vi "0MAIN_v1.vi"() -> ()   [LabVIEW 2021]
uses:
  <vilib>/Instr/_visa.llb/VISA Open Access Mode.ctl
  <vilib>/Instr/_visa.llb/VISA Configure Serial Port (Instr).vi
panel:
  out "LF2":bool
  out "LF1":bool
  out "Пересчитано":bool=TRUE
  out "Метка получена 2":bool
  out "Время старта":string
  out "Ошибка файла":errorcluster
  out "Метка получена":bool
  out "Файл данных":refnum<file>
  out "Файл журнала":refnum<file>
  out "Номер метки":bool=TRUE
  out "error out 2":errorcluster
  in  "Управление":enum32{"Отладка", "График", "Настройки"}(tab)
  in  "Пересчитать в частоты":bool
  in  "Частота метки 2":bool
  in  "Записать данные":bool
  in  "Очистка буфера":bool
  in  "Чтение данных":bool
  in  "Установить":string
  in  "Отправка":bool
  out "Данные с МК":string
  out "Развертка X (В/ГГц)":dbl[](array[numeric])
  out "Сигнал Y (В)":dbl[](array[numeric])
  out "Метки (В, ГГц)":dbl[][](array[numeric])
  in  "Частота метки":bool
  in  "Выход":bool
  in  "Расчет графика":bool
  out "График":T1(graph)
  in  "Путь к файлу данных":path
  in  "Путь к логу":path
  in  "Логирование":bool
  out "Ошибка":T2
  in  "Порт":refnum<visa-resource-name>
  in  "Скорость передачи (9600)":u32=9600
  in  "Символ окончания (\\n)":u8=10 format="%.0x"
  in  "Режим доступа":T3 items=["VISA Defaults"=0, "Exclusive Lock"=1, "Load Configured Settings"=4]
  in  "Бит данных (8)":u8=8 format="%.0x"
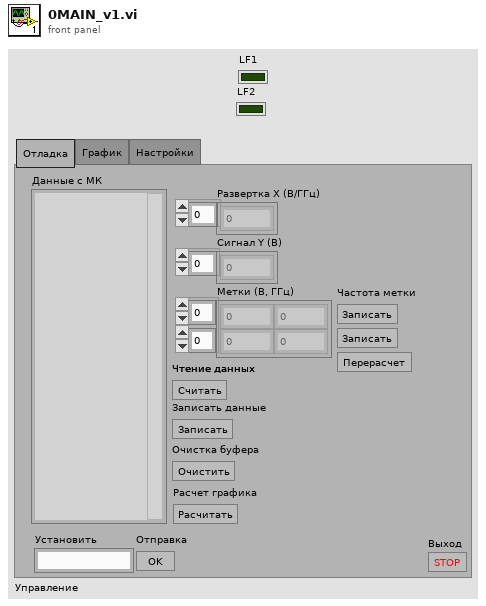
[diagram p1: front panel]
types:
  T1 = cluster{"Развертка X (В)":dbl[], "Сигнал Y (В)":dbl[]}
  T2 = cluster{"Статус":bool, "Код":i32, "Источник":string}
  T3 = typedef "VISA Open Access Mode.ctl" = u32
  T4 = enum16{"open", "replace", "create", "open or create", "replace or create", "replace or create with confirmation"}
  T5 = typedef "NI_Matrix.lvlib/RealMatrix.ctl" = dbl[][]
  T6 = cluster{"Развертка X (В/ГГц)":dbl[], "Сигнал Y (В)":dbl[]}
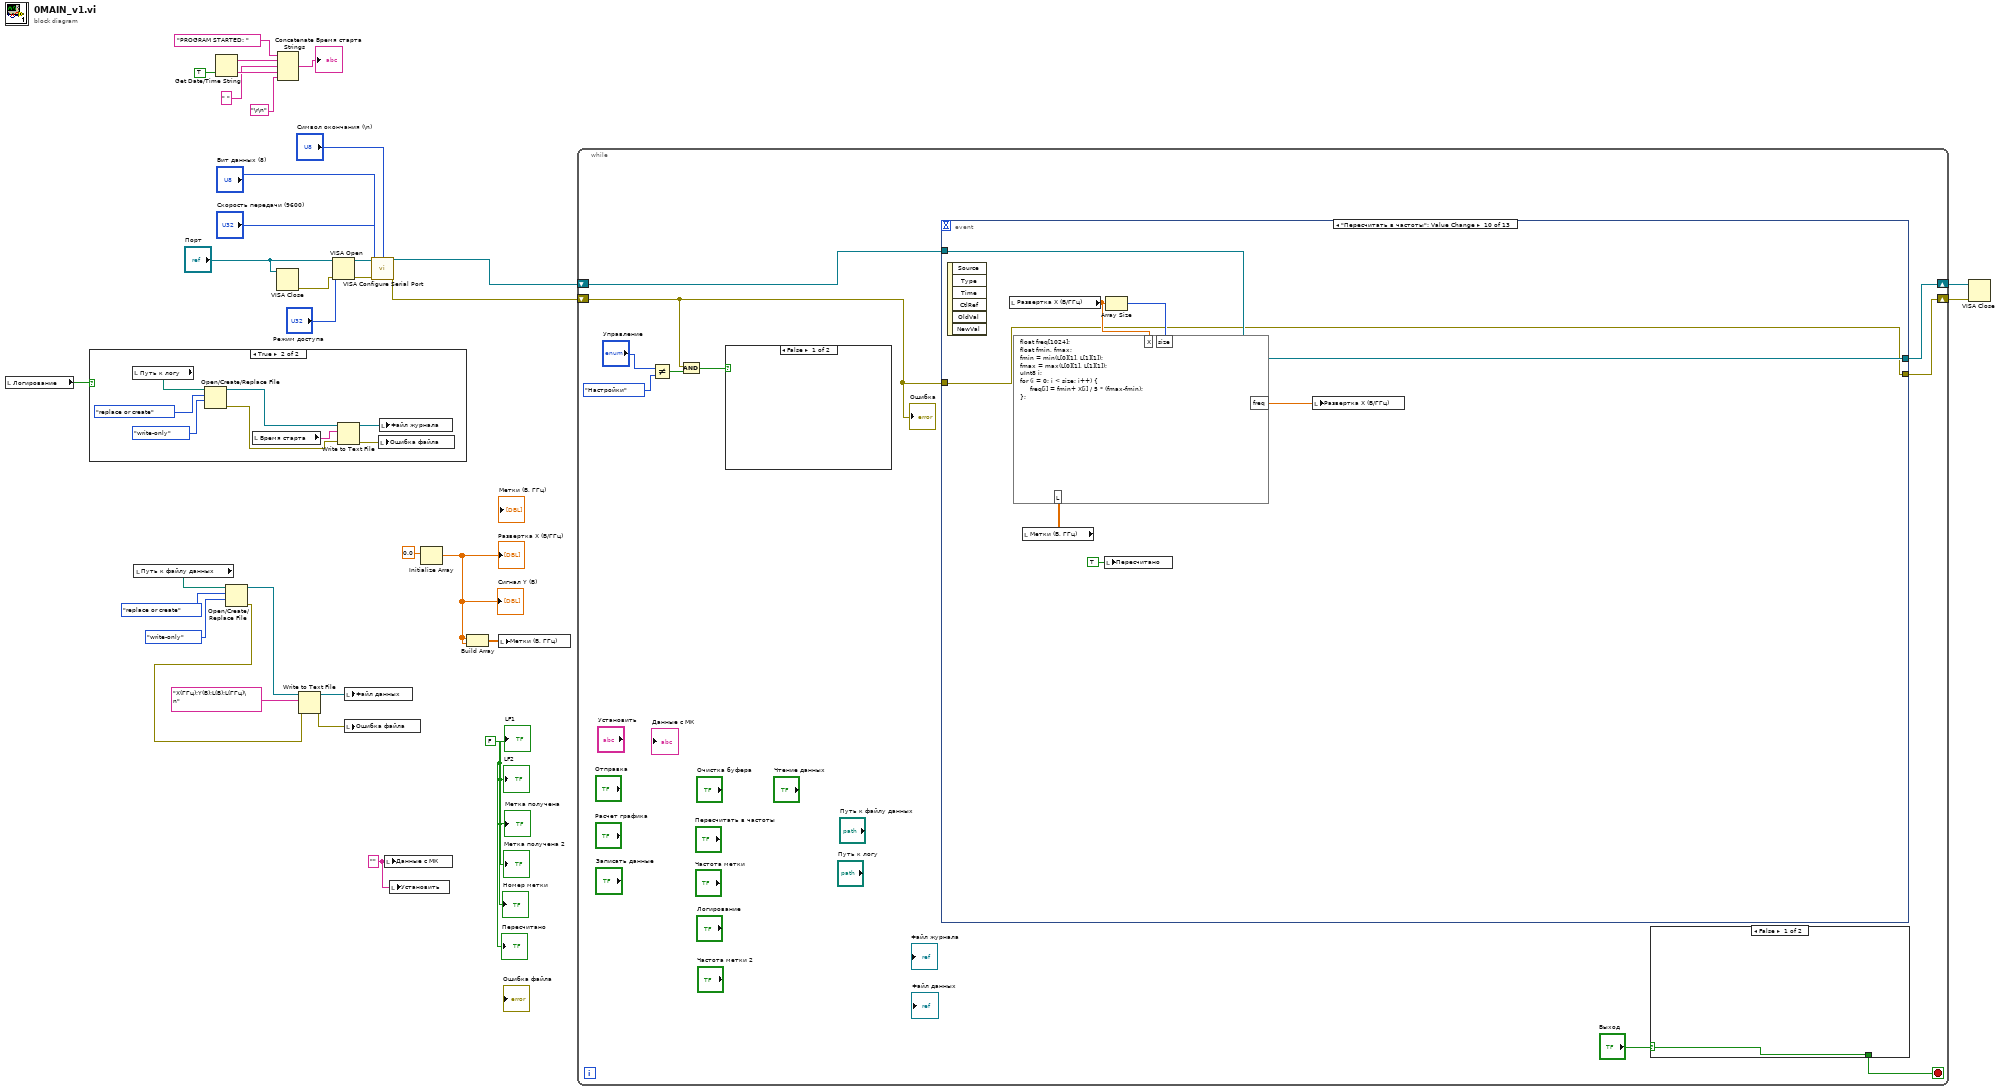
[diagram p0: block diagram]
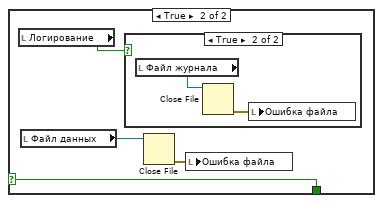
[diagram p3: hidden frame]
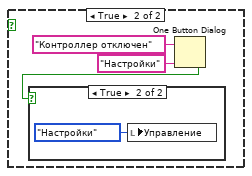
[diagram p5: hidden frame]
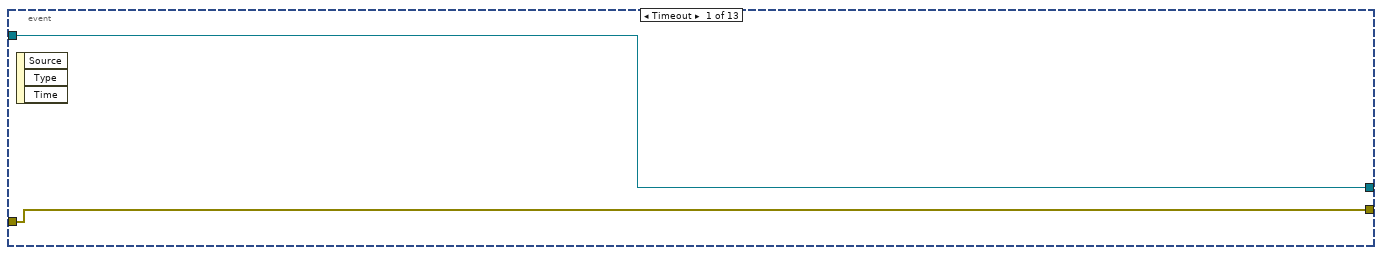
[diagram p7: hidden frame]
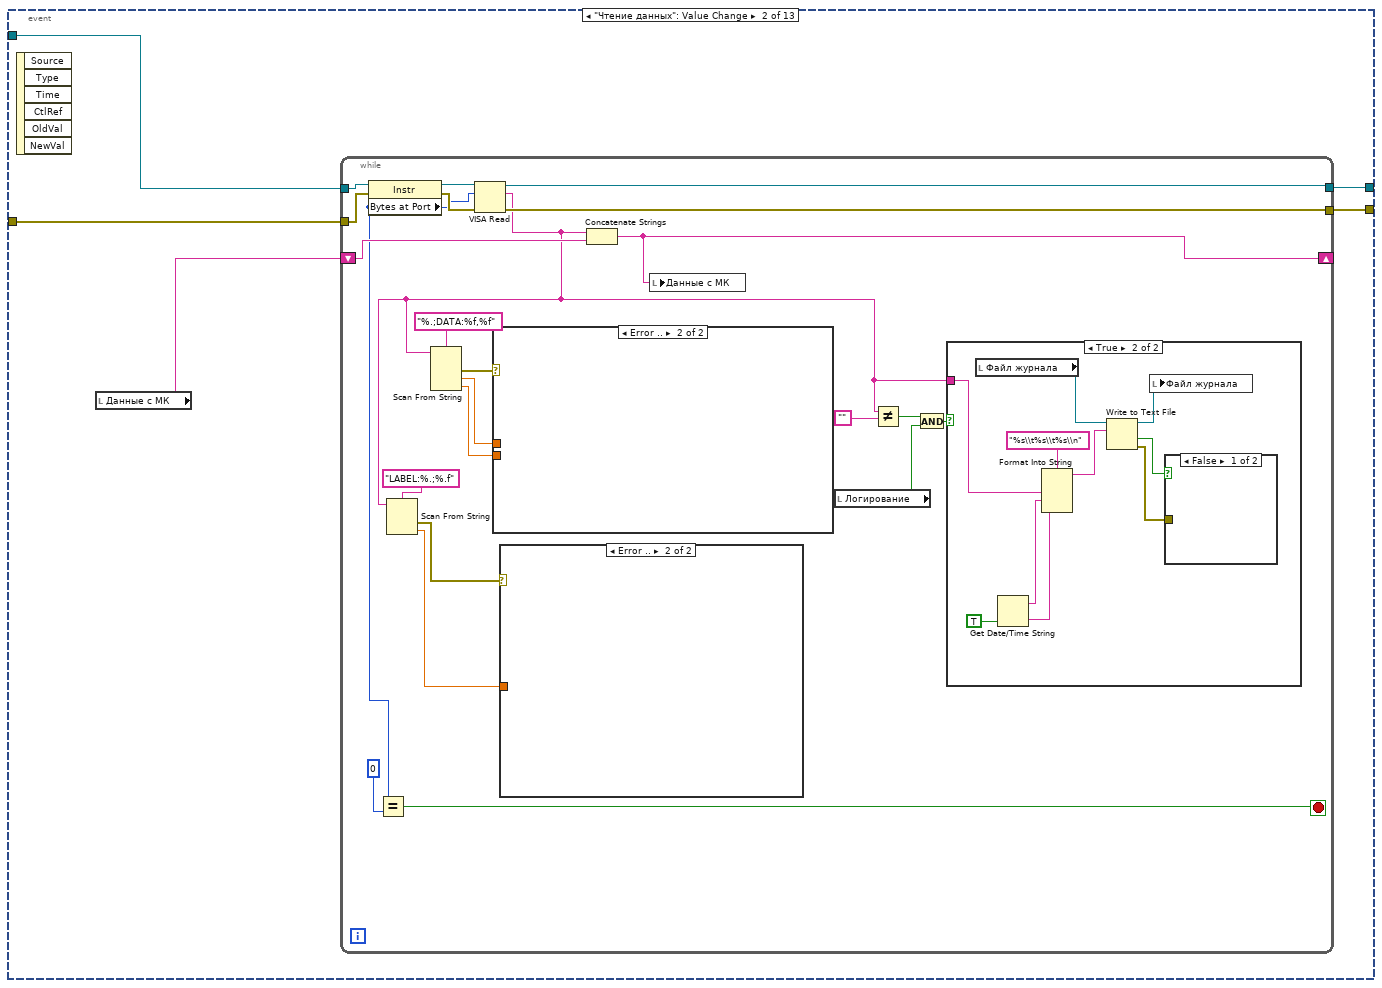
[diagram p8: hidden frame]
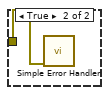
[diagram p10: hidden frame]
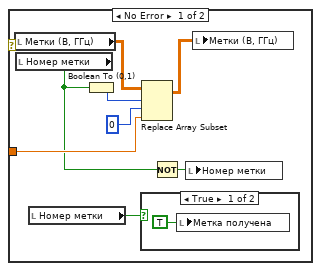
[diagram p11: hidden frame]
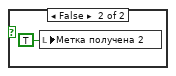
[diagram p12: hidden frame]
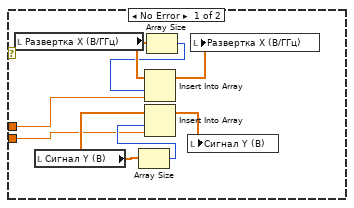
[diagram p13: hidden frame]
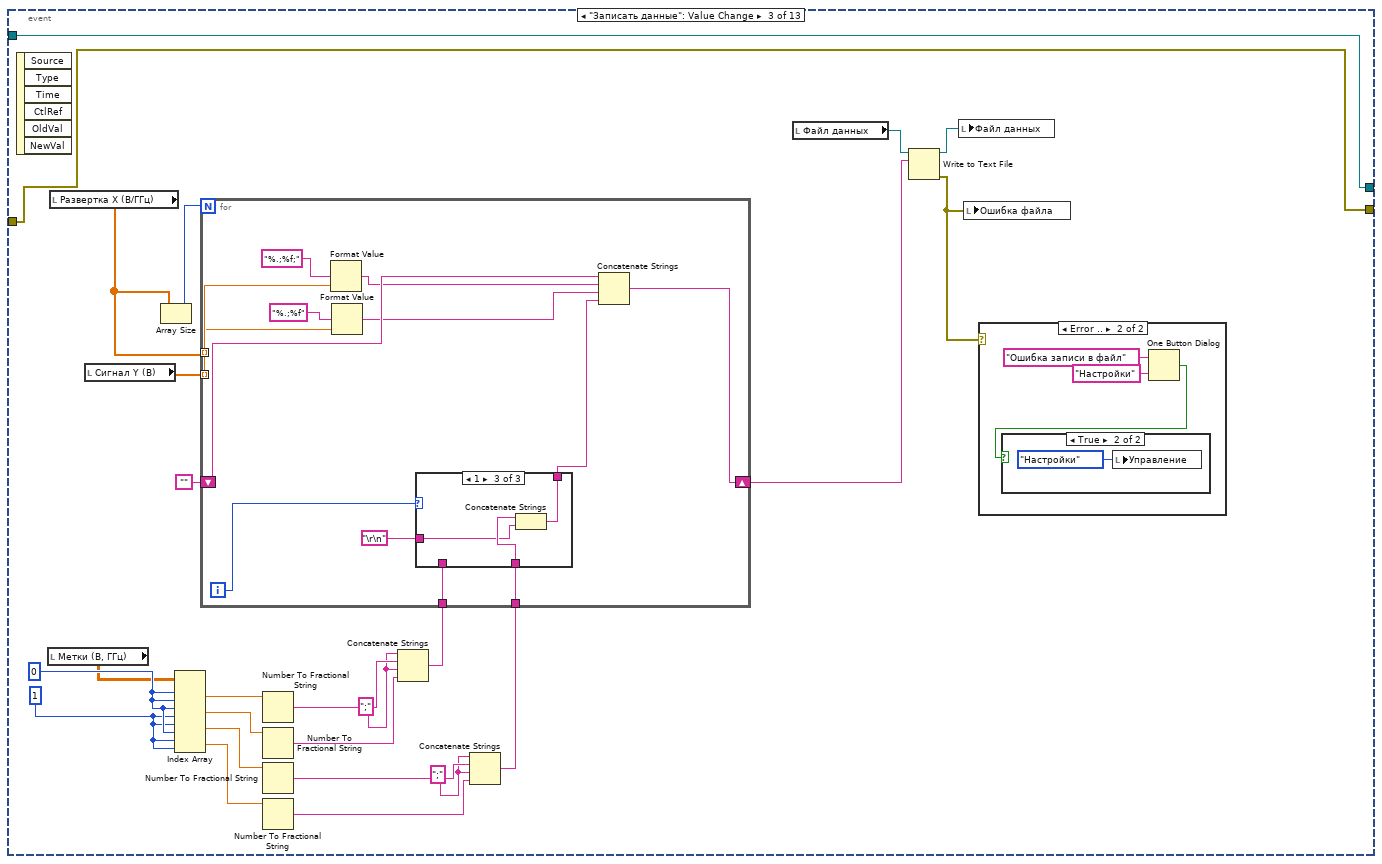
[diagram p14: hidden frame]
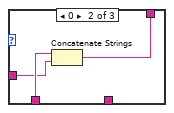
[diagram p18: hidden frame]
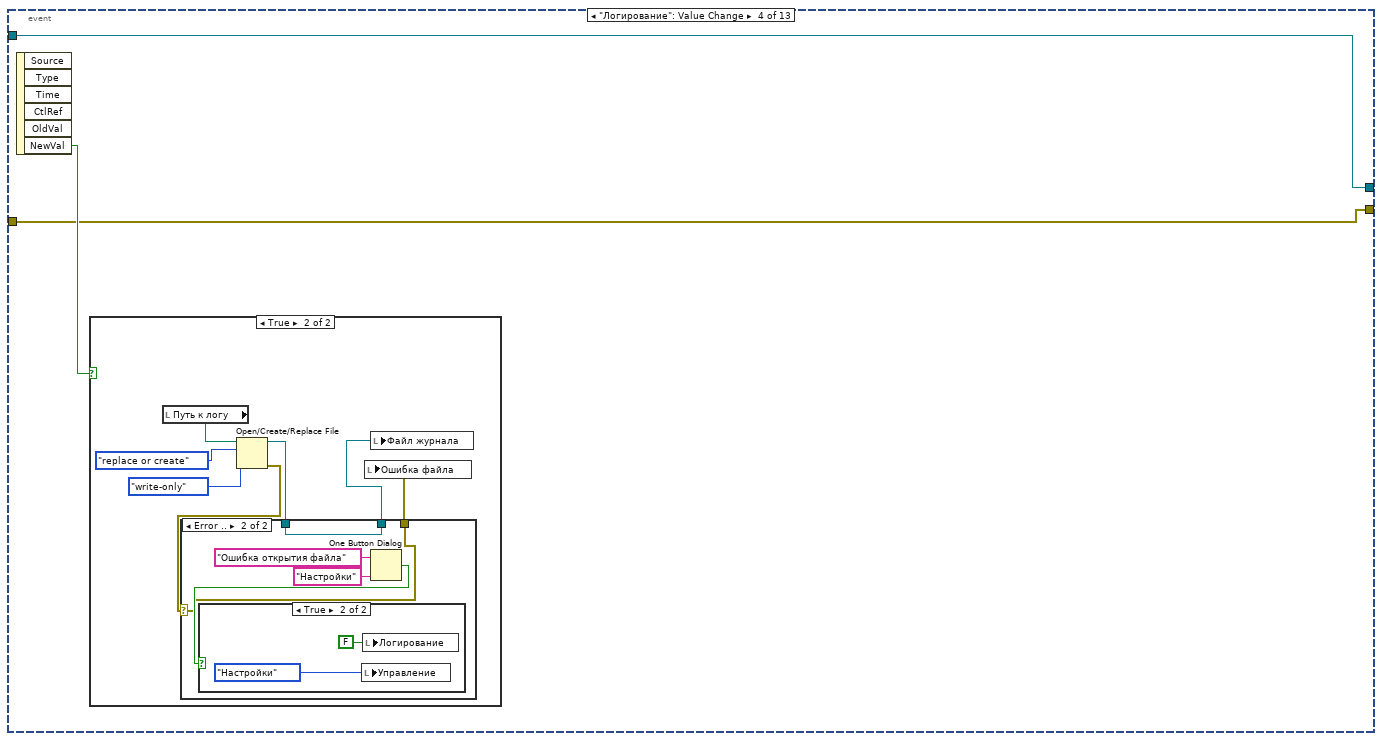
[diagram p19: hidden frame]
diagram:
  w1 = "" ("Данные с МК")
  w2 = FALSE ("Частоты определены")
  n1 = local read "Логирование"() -> (w13:bool)
  n2 = case shown="True" w13 {
    frame False {
    }
    frame True {
      n3 = local read "Путь к логу"() -> (w41:path)
      n4 = Open/Create/Replace File(file path (use dialog)=w41, operation (0:open)=T4."replace or create", access (0:read/write)=enum16{"read/write", "read-only", "write-only"}."write-only") -> (refnum out=w34:refnum<file>, error out=w35:errorcluster)  [unwired: 3 in, 1 out]
      n5 = local read "Время старта"() -> (w36:string)
      n6 = Write to Text File(file (use dialog)=w34, text=w36, error in=w35) -> (refnum out=w37:refnum<file>, error out=w38:errorcluster)  [unwired: 1 in, 1 out]
      n7 = local write "Ошибка файла"(w38) -> ()
      n8 = local write "Файл журнала"(w37) -> ()
    }
  }
  n9 = local read "Путь к файлу данных"() -> (w18:path)
  n10 = Get Date/Time String(want seconds? (F)=TRUE) -> (date string=w12:string, time string=w4:string)  [unwired: 2 in]
  n11 = Open/Create/Replace File(file path (use dialog)=w18, operation (0:open)=T4."replace or create", access (0:read/write)=enum16{"read/write", "read-only", "write-only"}."write-only") -> (refnum out=w6:refnum<file>, error out=w7:errorcluster)  [unwired: 3 in, 1 out]
  n12 = VISA Close(VISA resource name="Порт") -> (error out=w19:errorcluster)  [unwired: 1 in]
  n13 = Concatenate Strings("PROGRAM STARTED: " ("string"), w12, " ", w4, "\r\n" ("string")) -> (→"Время старта":string)
  n14 = Write to Text File(file (use dialog)=w6, text="X(ГГц);Y(В);L(В);L(ГГц)\n", error in=w7) -> (refnum out=w9:refnum<file>, error out=w10:errorcluster)  [unwired: 1 in, 1 out]
  n15 = VISA Open(access mode="Режим доступа", error in (no error)=w19, VISA resource name="Порт") -> (VISA resource name=w30:refnum<visa-resource-name>, error out=w29:errorcluster)  [unwired: 2 in]
  n16 = local write "Файл данных"(w9) -> ()
  n17 = local write "Ошибка файла"(w10) -> ()
  n18 = call-poly "VISA Configure Serial Port"("VISA resource name"=w30, "termination char\n(0xA = '\\n' = LF)"="Символ окончания (\\n)", "baud rate (9600)"="Скорость передачи (9600)", "data bits (8)"="Бит данных (8)", "error in (no error)"=w29) -> ("VISA resource name out"=w24:refnum<visa-resource-name>, "error out"=w26:errorcluster)  [unwired: 9 in]
  n19 = local write "Данные с МК"(w1) -> ()
  n20 = local write "Установить"(w1) -> ()
  n21 = Initialize Array(0.0 ("element")) -> (w21:dbl[])  [unwired: 1 in]
  "Развертка X (В/ГГц)" <- w21
  "Сигнал Y (В)" <- w21
  n22 = Build Array(w21, w21) -> (w20:T5)
  n23 = local write "Метки (В, ГГц)"(w20) -> ()
  n24 = while {
    shift-right: [w43] -> w25
    shift-left: w26 -> [w47]
    shift-right: [w42] -> w23
    shift-left: w24 -> [w51]
    stop <- w44 stop-if-true
    n25 = Not Equal?(x="Управление", y=enum32{"Отладка", "График", "Настройки"}."Настройки" ("Tab Control")) -> (x != y?=w48:bool)
    n26 = And(x=w47, y=w48) -> (x .and. y?=w46:bool)
    n27 = case shown="False" w46 {
      frame False {
      }
      frame True {
        n28 = One Button Dialog(message="Контроллер отключен", button name ("OK")="Настройки") -> (true=w60:bool)
        n29 = case shown="True" w60 {
          frame False {
          }
          frame True {
            n30 = local write "Управление"(enum32{"Отладка", "График", "Настройки"}."Настройки" ("Tab Control")) -> ()
          }
        }
      }
    }
    n31 = event shown="[9] \"Пересчитать в частоты\": Value Change" {
      selector: _ -> [_ _ _ _ _ _ _ _ _ _ _ _ _]
      dyn-events: _ -> [_ _ _ _ _ _ _ _ _ _ _ _ _]
      timeout: _ -> [_ _ _ _ _ _ _ _ _ _ _ _ _]
      tunnel: w47 -> [w64 w69 w122 w172 w193 _ w208 w218 w232 w237 w244 w269 w281]
      tunnel: [w64 w68 w122 w172 w193 w198 w208 w218 w232 w237 w244 w269 w280] -> w43
      tunnel: w51 -> [w63 w67 w123 w171 w194 _ w207 w219 w233 w238 w245 w270 w279]
      tunnel: [w63 w66 w123 w171 w194 w202 w207 w219 w233 w238 w245 w270 w278] -> w42
      event Timeout {
        n32 = event-data() -> ()  [unwired: 1 in, 3 out]
      }
      event "Чтение данных": Value Change {
        n33 = event-data() -> ()  [unwired: 1 in, 6 out]
        n34 = local read "Данные с МК"() -> (w65:string)
        n35 = while {
          tunnel: w67 -> [w87]
          tunnel: w69 -> [w86]
          tunnel: [w92] -> w66
          tunnel: [w91] -> w68
          shift-right: [w75] -> _
          shift-left: w65 -> [w90]
          stop <- w85 stop-if-true
          n36 = property class="Instr"(reference=w87, error in=w86) -> (reference out=w89:refnum<visa-resource-name>, error out=w88:errorcluster, "Bytes at Port"=w83:u32)
          n37 = Equal?(x=w83, y=u32 0 ("x")) -> (x = y?=w85:bool)
          n38 = VISA Read(VISA resource name=w89, byte count=w83, error in (no error)=w88) -> (VISA resource name out=w92:refnum<visa-resource-name>, read buffer=w71:string, error out=w91:errorcluster)  [unwired: 1 out]
          n39 = Scan From String(format string="LABEL:%.;%.f", input string=w71) -> (error out=w79:errorcluster, output 1=w78:dbl)  [unwired: 3 in, 2 out]
          n40 = Scan From String(format string="%.;DATA:%f,%f", input string=w71) -> (error out=w76:errorcluster, output 1=w82:dbl, output 2=w81:dbl)  [unwired: 4 in, 2 out]
          n41 = case shown="Error .." w76 {
            tunnel: w82 -> [w117 _]
            tunnel: w81 -> [w116 _]
            frame No Error {
              n42 = local read "Развертка X (В/ГГц)"() -> (w121:dbl[])
              n43 = local read "Сигнал Y (В)"() -> (w120:dbl[])
              n44 = Array Size(array=w120) -> (size(s)=w119:i32)
              n45 = Insert Into Array(array=w120, index=w119, new element=w116) -> (w114:dbl[])
              n46 = Array Size(array=w121) -> (size(s)=w118:i32)
              n47 = Insert Into Array(array=w121, index=w118, new element=w117) -> (w115:dbl[])
              n48 = local write "Сигнал Y (В)"(w114) -> ()
              n49 = local write "Развертка X (В/ГГц)"(w115) -> ()
            }
            frame Error {
            }
          }
          n50 = case shown="Error .." w79 {
            tunnel: w78 -> [w108 _]
            frame No Error {
              n51 = local read "Метки (В, ГГц)"() -> (w110:dbl[][])
              n52 = local read "Номер метки"() -> (w105:bool)
              n53 = local read "Номер метки"() -> (w104:bool)
              n54 = Boolean To (0,1)(Boolean=w105) -> (0, 1=w109:i16)
              n55 = case shown="True" w104 {
                frame True {
                  n56 = local write "Метка получена"(TRUE ("Метка получена")) -> ()
                }
                frame False {
                  n57 = local write "Метка получена 2"(TRUE ("Метка получена")) -> ()
                }
              }
              n58 = Replace Array Subset(array=w110, new element=w108, index (row)=w109, index (col)=0 ("disabled index (col)")) -> (w111:T5)
              n59 = Not(x=w105) -> (.not. x?=w106:bool)
              n60 = local write "Номер метки"(w106) -> ()
              n61 = local write "Метки (В, ГГц)"(w111) -> ()
            }
            frame Error {
            }
          }
          n62 = Concatenate Strings(w71, w90) -> (w75:string)
          n63 = local write "Данные с МК"(w75) -> ()
          n64 = local read "Логирование"() -> (w70:bool)
          n65 = Not Equal?(x=w71, y="") -> (x != y?=w73:bool)
          n66 = And(x=w73, y=w70) -> (x .and. y?=w74:bool)
          n67 = case shown="True" w74 {
            tunnel: w71 -> [_ w93]
            frame False {
            }
            frame True {
              n68 = local read "Файл журнала"() -> (w98:refnum<file>)
              n69 = Get Date/Time String(want seconds? (F)=TRUE) -> (date string=w97:string, time string=w96:string)  [unwired: 2 in]
              n70 = Format Into String(format string="%s\\t%s\\t%s\\n", w93, w97, w96) -> (resulting string=w94:string)  [unwired: 2 in, 1 out]
              n71 = Write to Text File(file (use dialog)=w98, text=w94) -> (refnum out=w99:refnum<file>, cancelled=w101:bool, error out=w100:errorcluster)  [unwired: 2 in]
              n72 = local write "Файл журнала"(w99) -> ()
              n73 = case shown="False" w101 {
                tunnel: w100 -> [_ w103]
                frame False {
                }
                frame True {
                  n74 = call <vilib>:"Simple Error Handler.vi"("error in (no error)"=w103) -> ()  [unwired: 4 in, 5 out]
                }
              }
            }
          }
        }
      }
      event "Записать данные": Value Change {
        w128 = ";"
        w129 = ";"
        w140 = 1
        w141 = 0
        n75 = event-data() -> ()  [unwired: 1 in, 6 out]
        n76 = local read "Метки (В, ГГц)"() -> (w127:dbl[][])
        n77 = local read "Развертка X (В/ГГц)"() -> (w144:dbl[])
        n78 = local read "Сигнал Y (В)"() -> (w145:dbl[])
        n79 = Array Size(array=w144) -> (size(s)=w146:i32)
        n80 = Index Array(array=w127, index (row) #1=w141, index (col) #1=w141, index (row) #2=w141, index (col) #2=w140, index (row) #3=w140, index (col) #3=w141, index (row) #4=w140, index (col) #4=w140) -> (element #1=w139:dbl, element #2=w138:dbl, element #3=w137:dbl, element #4=w136:dbl)
        n81 = Number To Fractional String(number=w139) -> (F-format string=w132:string)  [unwired: 3 in]
        n82 = Number To Fractional String(number=w138) -> (F-format string=w133:string)  [unwired: 3 in]
        n83 = Number To Fractional String(number=w137) -> (F-format string=w134:string)  [unwired: 3 in]
        n84 = Number To Fractional String(number=w136) -> (F-format string=w135:string)  [unwired: 3 in]
        n85 = Concatenate Strings(w128, w132, w128, w133) -> (w131:string)
        n86 = Concatenate Strings(w129, w134, w129, w135) -> (w130:string)
        n87 = for {
          N: w146 -> [_]
          tunnel: w145 -> [w162] mode=indexing
          tunnel: w144 -> [w163] mode=indexing
          shift-right: [w159] -> w126
          shift-left: "" -> [w154]
          tunnel: w131 -> [w157]
          tunnel: w130 -> [w156]
          i -> [w158]
          n88 = Format Value(format string="%.;%f;", value (0)=w163) -> (output string=w153:string)  [unwired: 1 in]
          n89 = Format Value(format string="%.;%f", value (0)=w162) -> (output string=w152:string)  [unwired: 1 in]
          n90 = case shown="1" w158 {
            tunnel: w157 -> [_ w167 _]
            tunnel: w156 -> [_ _ w170]
            tunnel: "\r\n" -> [w164 w166 w169]
            tunnel: [w164 w165 w168] -> w151
            frame Default {
            }
            frame 0 {
              n91 = Concatenate Strings(w167, w166) -> (w165:string)
            }
            frame 1 {
              n92 = Concatenate Strings(w170, w169) -> (w168:string)
            }
          }
          n93 = Concatenate Strings(w154, w153, w152, w151) -> (w159:string)
        }
        n94 = local read "Файл данных"() -> (w143:refnum<file>)
        n95 = Write to Text File(file (use dialog)=w143, text=w126) -> (refnum out=w142:refnum<file>, error out=w124:errorcluster)  [unwired: 2 in, 1 out]
        n96 = local write "Файл данных"(w142) -> ()
        n97 = local write "Ошибка файла"(w124) -> ()
        n98 = case shown="Error .." w124 {
          frame No Error {
          }
          frame Error {
            n99 = One Button Dialog(message="Ошибка записи в файл", button name ("OK")="Настройки") -> (true=w148:bool)
            n100 = case shown="True" w148 {
              frame False {
              }
              frame True {
                n101 = local write "Управление"(enum32{"Отладка", "График", "Настройки"}."Настройки" ("Управление")) -> ()
              }
            }
          }
        }
      }
      event "Логирование": Value Change {
        n102 = event-data() -> ("NewVal"=w173:bool)  [unwired: 1 in, 5 out]
        n103 = case shown="True" w173 {
          frame False {
          }
          frame True {
            n104 = local read "Путь к логу"() -> (w180:path)
            n105 = Open/Create/Replace File(file path (use dialog)=w180, operation (0:open)=T4."replace or create", access (0:read/write)=enum16{"read/write", "read-only", "write-only"}."write-only") -> (refnum out=w178:refnum<file>, error out=w179:errorcluster)  [unwired: 3 in, 1 out]
            n106 = case shown="Error .." w179 {
              selector: w179 -> [w184 w186]
              tunnel: w178 -> [w185 w187]
              tunnel: [w183 w186] -> w177
              tunnel: [w182 w187] -> w176
              frame No Error {
                n107 = local read "Время старта"() -> (w181:string)
                n108 = Write to Text File(file (use dialog)=w185, text=w181, error in=w184) -> (refnum out=w182:refnum<file>, error out=w183:errorcluster)  [unwired: 1 in, 1 out]
              }
              frame Error {
                n109 = One Button Dialog(message="Ошибка открытия файла", button name ("OK")="Настройки") -> (true=w189:bool)
                n110 = case shown="True" w189 {
                  frame False {
                  }
                  frame True {
                    n111 = local write "Управление"(enum32{"Отладка", "График", "Настройки"}."Настройки" ("Управление")) -> ()
                    n112 = local write "Логирование"(FALSE ("Логирование")) -> ()
                  }
                }
              }
            }
            n113 = local write "Ошибка файла"(w177) -> ()
            n114 = local write "Файл журнала"(w176) -> ()
          }
        }
      }
      event "Очистка буфера": Value Change {
        n115 = event-data() -> ()  [unwired: 1 in, 6 out]
        n116 = local write "Данные с МК"("") -> ()
      }
      event "Порт": Value Change {
        n117 = event-data() -> ("OldVal"=w197:refnum<visa-resource-name>, "NewVal"=w206:refnum<visa-resource-name>)  [unwired: 1 in, 4 out]
        n118 = local read "Скорость передачи (9600)"() -> (w201:u32)
        n119 = local read "Бит данных (8)"() -> (w200:u8)
        n120 = local read "Режим доступа"() -> (w205:T3)
        n121 = local read "Символ окончания (\\n)"() -> (w199:u8)
        n122 = VISA Close(VISA resource name=w197) -> (error out=→"error out 2":errorcluster)  [unwired: 1 in]
        n123 = VISA Open(access mode=w205, VISA resource name=w206) -> (VISA resource name=w204:refnum<visa-resource-name>, error out=w203:errorcluster)  [unwired: 3 in]
        n124 = call-poly "VISA Configure Serial Port"("VISA resource name"=w204, "termination char\n(0xA = '\\n' = LF)"=w199, "baud rate (9600)"=w201, "data bits (8)"=w200, "error in (no error)"=w203) -> ("VISA resource name out"=w202:refnum<visa-resource-name>, "error out"=w198:errorcluster)  [unwired: 9 in]
      }
      event "Частота метки": Value Change {
        n125 = event-data() -> ()  [unwired: 1 in, 6 out]
        n126 = local read "Метка получена"() -> (w209:bool)
        n127 = case shown="True" w209 {
          frame False {
          }
          frame True {
            n128 = local read "Установить"() -> (w216:string)
            n129 = local read "Метки (В, ГГц)"() -> (w212:dbl[][])
            n130 = Scan Value(string=w216, format string="%.;%f") -> (value=w217:dbl)  [unwired: 1 in, 1 out]
            n131 = Replace Array Subset(array=w212, new element=w217, index (row)=0 ("disabled index (row)"), index (col)=1 ("disabled index (col)")) -> (w213:T5)
            n132 = local write "Метки (В, ГГц)"(w213) -> ()
            n133 = local write "LF1"(TRUE ("LF1")) -> ()
          }
        }
      }
      event "Частота метки 2": Value Change {
        n134 = event-data() -> ()  [unwired: 1 in, 6 out]
        n135 = local read "Метка получена 2"() -> (w220:bool)
        n136 = case shown="True" w220 {
          frame False {
          }
          frame True {
            n137 = local read "Установить"() -> (w227:string)
            n138 = local read "Метки (В, ГГц)"() -> (w223:dbl[][])
            n139 = Scan Value(string=w227, format string="%.;%f") -> (value=w228:dbl)  [unwired: 1 in, 1 out]
            n140 = Replace Array Subset(array=w223, new element=w228, index (row)=1 ("disabled index (row)"), index (col)=1 ("disabled index (col)")) -> (w224:T5)
            n141 = local write "Метки (В, ГГц)"(w224) -> ()
            n142 = local write "LF2"(TRUE ("LF2")) -> ()
          }
        }
      }
      event "Расчет графика": Value Change {
        n143 = event-data() -> ()  [unwired: 1 in, 6 out]
        n144 = local read "Пересчитано"() -> (w229:bool)
        n145 = local read "Развертка X (В/ГГц)"() -> (w231:dbl[])
        n146 = local read "Сигнал Y (В)"() -> (w234:dbl[])
        n147 = case shown="False" w229 {
          frame False {
            n148 = property on="График" class="XYGraph (strict)"("XScale.NameLbl.Text"="Развертка Х, В" ("X Scale.Name Label.Text")) -> ()  [unwired: 2 in, 2 out]
          }
          frame True {
            n149 = property on="График" class="XYGraph (strict)"("XScale.NameLbl.Text"="Частота Х, ГГц" ("X Scale.Name Label.Text")) -> ()  [unwired: 2 in, 2 out]
          }
        }
        n150 = Bundle("Развертка X (В/ГГц)"=w231, "Сигнал Y (В)"=w234) -> (→"График":T6)  [unwired: 1 in]
      }
      event "Пересчитать в частоты": Value Change {
        n151 = event-data() -> ()  [unwired: 1 in, 6 out]
        n152 = local read "Развертка X (В/ГГц)"() -> (w242:dbl[])
        n153 = local read "Метки (В, ГГц)"() -> (w241:dbl[][])
        n154 = local write "Пересчитано"(TRUE ("Пересчитано")) -> ()
        n155 = Array Size(array=w242) -> (size(s)=w243:i32)
        n156 = formula code="float freq[1024];\nfloat fmin, fmax;\nfmin = min(L[0][1], L[1][1]);\nfmax = max(L[0][1], L[1][1]);\nuInt8 i;\nfor (i = 0; i < size; i++) {\n     freq[i] = fmin+ X[i] / 5 * (fmax-fmin);\n};"("L"=w241, "X"=w242, "size"=w243) -> ("freq"=w240:dbl[])
        n157 = local write "Развертка X (В/ГГц)"(w240) -> ()
      }
      event "Путь к логу": Value Change {
        n158 = event-data() -> ("NewVal"=w246:path)  [unwired: 1 in, 5 out]
        n159 = local read "Логирование"() -> (w248:bool)
        n160 = case shown="True" w248 {
          selector: w248 -> [w257 w258]
          tunnel: [w257 w258] -> w247
          frame False {
          }
          frame True {
            n161 = local read "Файл журнала"() -> (w259:refnum<file>)
            n162 = Close File(refnum=w259) -> ()  [unwired: 1 in, 2 out]
          }
        }
        n163 = case shown="True" w247 {
          tunnel: w246 -> [_ w254]
          frame False {
          }
          frame True {
            n164 = local read "Время старта"() -> (w252:string)
            n165 = Open/Create/Replace File(file path (use dialog)=w254, operation (0:open)=T4."replace or create", access (0:read/write)=enum16{"read/write", "read-only", "write-only"}."write-only") -> (refnum out=w249:refnum<file>, error out=w251:errorcluster)  [unwired: 3 in, 1 out]
            n166 = Write to Text File(file (use dialog)=w249, text=w252, error in=w251) -> (refnum out=w250:refnum<file>, error out=w253:errorcluster)  [unwired: 1 in, 1 out]
            n167 = local write "Файл журнала"(w250) -> ()
            n168 = local write "Ошибка файла"(w253) -> ()
          }
        }
      }
      event "Путь к файлу данных": Value Change {
        n169 = event-data() -> ("NewVal"=w266:path)  [unwired: 1 in, 5 out]
        n170 = local read "Файл данных"() -> (w271:refnum<file>)
        n171 = Close File(refnum=w271) -> (error out=w260:errorcluster)  [unwired: 1 in, 1 out]
        n172 = local write "Ошибка файла"(w260) -> ()
        n173 = Open/Create/Replace File(file path (use dialog)=w266, operation (0:open)=T4."replace or create", access (0:read/write)=enum16{"read/write", "read-only", "write-only"}."write-only") -> (refnum out=w262:refnum<file>, error out=w264:errorcluster)  [unwired: 3 in, 1 out]
        n174 = Write to Text File(file (use dialog)=w262, text="X(ГГц);Y(В);L(В);L(ГГц)\n", error in=w264) -> (refnum out=w261:refnum<file>, error out=w263:errorcluster)  [unwired: 1 in, 1 out]
        n175 = local write "Файл данных"(w261) -> ()
        n176 = local write "Ошибка файла"(w263) -> ()
      }
      event "Отправка": Value Change {
        n177 = event-data() -> ()  [unwired: 1 in, 6 out]
        n178 = local read "Установить"() -> (w277:string)
        n179 = Scan From String(format string="%d,%s", input string=w277) -> (error out=w272:errorcluster, output 1=w275:i32, output 2=w274:string)  [unwired: 4 in, 2 out]
        n180 = local write "error out 2"(w272) -> ()
        n181 = case shown="4" w275 {
          tunnel: w274 -> [_ w290 w301 _ _]
          tunnel: ["" w285 w299 "02" "03"] -> w273
          frame 0, Default {
          }
          frame 1 {
            n182 = local read "LF1"() -> (w287:bool)
            n183 = local read "LF2"() -> (w286:bool)
            n184 = Scan From String(format string="%.;%f,%f", input string=w290) -> (output 1=w284:dbl, output 2=w283:dbl)  [unwired: 4 in, 3 out]
            n185 = And(x=w287, y=w286) -> (x .and. y?=w288:bool)
            n186 = case shown="True" w288 {
              tunnel: ["" w292] -> w285
              tunnel: w284 -> [_ w297]
              tunnel: w283 -> [_ w296]
              frame False {
              }
              frame True {
                n187 = local read "Метки (В, ГГц)"() -> (w298:dbl[][])
                n188 = formula code="float fmin = min(L[0][1],L[1][1]);\nfloat fmax = max(L[0][1],L[1][1]);\nu1 = (f1-fmin) / (fmax-fmin) * 5;\nu2 = (f2-fmin) / (fmax-fmin) * 5;"("L"=w298, "f1"=w297, "f2"=w296) -> ("u1"=w294:dbl, "u2"=w293:dbl)
                n189 = Format Into String(format string="%.;01,%.2f,%.2f", w294, w293) -> (resulting string=w292:string)  [unwired: 2 in, 1 out]
              }
            }
          }
          frame 4 {
            n190 = local read "LF1"() -> (w304:bool)
            n191 = local read "LF2"() -> (w303:bool)
            n192 = Scan From String(format string="%.;%f", input string=w301) -> (output 1=w300:dbl)  [unwired: 3 in, 3 out]
            n193 = And(x=w304, y=w303) -> (x .and. y?=w305:bool)
            n194 = case shown="True" w305 {
              tunnel: w300 -> [_ w310]
              tunnel: ["" w307] -> w299
              frame False {
              }
              frame True {
                n195 = local read "Метки (В, ГГц)"() -> (w311:dbl[][])
                n196 = formula code="float fmin = min(L[0][1],L[1][1]);\nfloat fmax = max(L[0][1],L[1][1]);\nu = (f-fmin) / (fmax-fmin) * 5;"("L"=w311, "f"=w310) -> ("u"=w308:dbl)
                n197 = Format Into String(format string="%.;04,%.2f", w308) -> (resulting string=w307:string)  [unwired: 2 in, 1 out]
              }
            }
          }
          frame 2 {
            n198 = Initialize Array(0.0 ("element")) -> (w313:dbl[])  [unwired: 1 in]
            n199 = local write "Развертка X (В/ГГц)"(w313) -> ()
            n200 = local write "Сигнал Y (В)"(w313) -> ()
            n201 = property on="График" class="XYGraph (strict)"("Plot.Plot Name"="КСВН") -> ()  [unwired: 2 in, 2 out]
          }
          frame 3 {
            n202 = Initialize Array(0.0 ("element")) -> (w318:dbl[])  [unwired: 1 in]
            n203 = local write "Развертка X (В/ГГц)"(w318) -> ()
            n204 = local write "Сигнал Y (В)"(w318) -> ()
            n205 = property on="График" class="XYGraph (strict)"("Plot.Plot Name"="Метка") -> ()  [unwired: 2 in, 2 out]
          }
        }
        n206 = VISA Write(VISA resource name=w279, write buffer=w273, error in (no error)=w281) -> (VISA resource name out=w278:refnum<visa-resource-name>, error out=w280:errorcluster)  [unwired: 1 out]
      }
    }
    n207 = case shown="False" "Выход" {
      selector: "Выход" -> [w52 w54]
      tunnel: [w52 w54] -> w44
      frame False {
      }
      frame True {
        n208 = local read "Логирование"() -> (w56:bool)
        n209 = local read "Файл данных"() -> (w55:refnum<file>)
        n210 = case shown="True" w56 {
          frame False {
          }
          frame True {
            n211 = local read "Файл журнала"() -> (w58:refnum<file>)
            n212 = Close File(refnum=w58) -> (error out=w57:errorcluster)  [unwired: 1 in, 1 out]
            n213 = local write "Ошибка файла"(w57) -> ()
          }
        }
        n214 = Close File(refnum=w55) -> (error out=w53:errorcluster)  [unwired: 1 in, 1 out]
        n215 = local write "Ошибка файла"(w53) -> ()
      }
    }
    "Ошибка" <- w47
  }
  n216 = VISA Close(VISA resource name=w23, error in (no error)=w25) -> ()  [unwired: 1 out]
  "Номер метки" <- w2
  "Метка получена" <- w2
  "Метка получена 2" <- w2
  "Пересчитано" <- w2
  "LF1" <- w2
  "LF2" <- w2
